vi "getViVersion.vi"(8 "error in (no error)":errorcluster, 11 "VI in":refnum<vi>) -> (0 "error out":errorcluster, 2 "Version":T1, 3 "VI out":refnum<vi>)   [LabVIEW 2017, in "vi_tools.lvlib"]
doc: "Returns the version information for the specified VI reference."
uses:
  vi_tools.lvlib
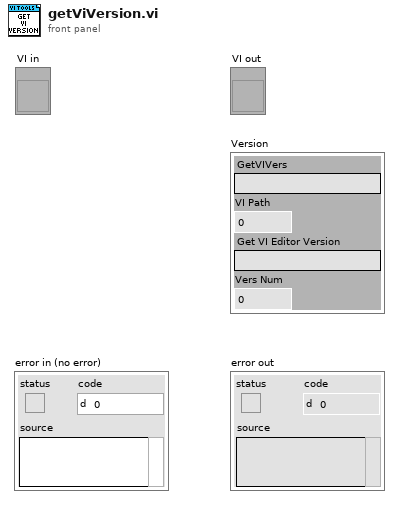
[diagram p1: front panel]
types:
  T1 = cluster{"GetVIVers":string, "VI Path":u32, "Get VI Editor Version":string, "Vers Num":u32}
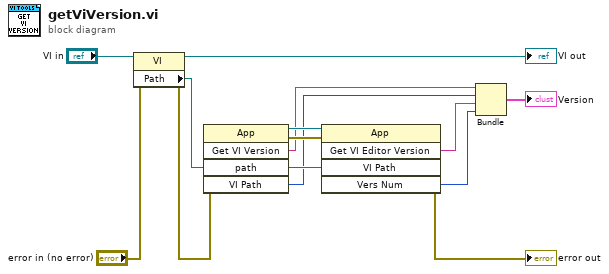
[diagram p0: block diagram]
diagram:
  n1 = property class="VI"(reference="VI in", error in="error in (no error)") -> (reference out=→"VI out":refnum<vi>, error out=w11:errorcluster, "Path"=w10:path)
  n2 = invoke class="App" method="Get VI Version"(error in=w11, "path"=w10) -> (reference out=w6:refnum<vi>, error out=w7:errorcluster, "GetVIVers"=w3:string, "VI Path"=w2:u32)  [unwired: 3 in, 1 out]
  n3 = invoke class="App" method="Get VI Editor Version"(reference=w6, error in=w7, "VI Path"=w10) -> (error out=→"error out":errorcluster, "Get VI Editor Version"=w5:string, "Vers Num"=w4:u32)  [unwired: 2 in, 2 out]
  n4 = Bundle("GetVIVers"=w3, "VI Path"=w2, "Get VI Editor Version"=w5, "Vers Num"=w4) -> (→"Version":T1)  [unwired: 1 in]
